vi "demo.vi"(0 "reference (in)":refnum<class "_Controller.lvclass">, 1 "position ref":refnum<vi>, 2 "position (large) ref":refnum<vi>, 5 "positions":i32[](array[numeric]), 11 "error in (no error)":errorcluster, 12 "status (display) ref":refnum<vi>, 13 "status ref":refnum<vi>) -> (4 "reference (out)":refnum<class "_Controller.lvclass">, 15 "error out":errorcluster)   [LabVIEW 2013, in "common.lvlib"]
doc: "Cycles the motor to each position in the input array of positions.\n\nProduced By:\n\n<B>Kod Integrations, LLC</B>\n4835 Marianne Drive\nMount Airy, MD 21771\nhttp://www.kodintegrations.com\nemail: info@kodintegrations.com\nphone: (240) 687-1288"
uses:
  libraries/common.lvlib
  controls/motor_status.ctl
  classes/Controller/_Controller.lvclass
  controls/axis.ctl
  controls/movement_item.ctl
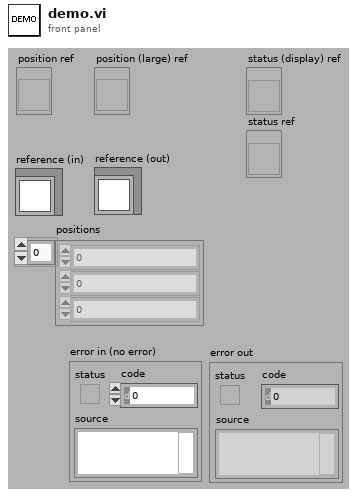
[diagram p1: front panel]
types:
  T1 = typedef "common.lvlib/movement_item.ctl" = cluster{"axis":T2, "target":i32}
  T2 = typedef "common.lvlib/axis.ctl" = enum16{"X", "Y", "Z", "U"}
  T3 = typedef "common.lvlib/motor_status.ctl" = enum16{"IDLE", "CONST", "ACCEL", "DECEL", "HOME_SWITCH", "-LIMIT_SWITCH", "+LIMIT_SWITCH", "-LIMIT_ERR", "+LIMIT_ERR", "COMM_TIMEOUT", "ALARM_INPUT", "ALARM_ERROR", "TOC_TIMEOUT_STATUS", "LATCH_INPUT_STATUS", "Z_INDEX_STATUS"}
  T4 = typedef "common.lvlib/complete_motor_state.ctl" = cluster{"X":T5, "Y":T5, "Z":T5, "U":T5, "buffer_enabled?":bool, "buffer_start":i32, "buffer_end":i32, "avail_buffer":i32, "move_mode":T6}
  T5 = typedef "common.lvlib/single_axis_state.ctl" = cluster{"motion_state":T3, "other_states":T3[]}
  T6 = typedef "common.lvlib/move_mode.ctl" = enum16{"ABSOLUTE", "INCREMENTAL"}
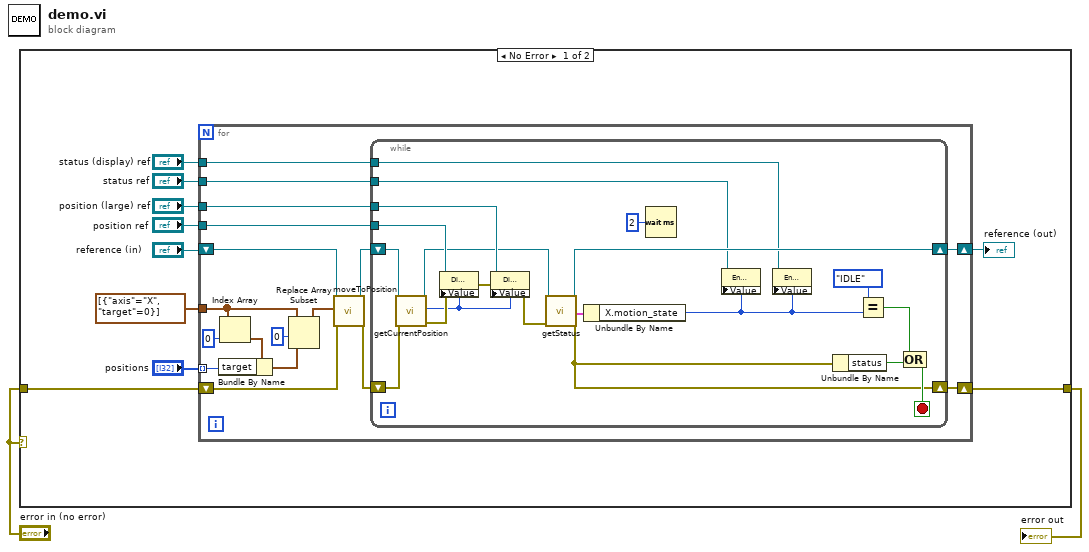
[diagram p0: block diagram]
diagram:
  n1 = case shown="No Error" "error in (no error)" {
    tunnel: "error in (no error)" -> [w8 w50]
    tunnel: [w7 w50] -> w1
    frame No Error {
      n2 = for {
        shift-right: [w23] -> w7
        shift-left: w8 -> [w24]
        tunnel: "positions" -> [w17] mode=indexing
        shift-right: [w27] -> w9
        shift-left: "reference (in)" -> [w29]
        tunnel: "position ref" -> [w26]
        tunnel: "position (large) ref" -> [w22]
        tunnel: "status (display) ref" -> [w21]
        tunnel: "status ref" -> [w20]
        tunnel: T1[] [{"axis"=enum."X", "target"=0}] ("target(s) (in)") -> [w16]
        n3 = Index Array(array=w16, index=0) -> (element=w18:T1)
        n4 = Bundle By Name(cluster=w18, "target"=w17) -> (w14:T1)
        n5 = Replace Array Subset(array=w16, new element=w14, index=0) -> (w13:T1[])
        n6 = call-dynamic "moveToPosition.vi"("Controller in"=w29, "target(s) (in)"=w13, "error in (no error)"=w24) -> ("Controller out"=w28:refnum<class "_Controller.lvclass">, "error out"=w25:errorcluster)  [unwired: 13 in, 2 out]
        n7 = while {
          shift-right: [w48] -> w27
          shift-left: w28 -> [w42]
          tunnel: w26 -> [w45]
          shift-right: [w41] -> w23
          shift-left: w25 -> [w44]
          tunnel: w22 -> [w39]
          tunnel: w21 -> [w36]
          tunnel: w20 -> [w35]
          stop <- w46 stop-if-true
          n8 = call-dynamic "getCurrentPosition.vi"("reference (in)"=w42, "error in (no error)"=w44) -> ("reference (out)"=w34:refnum<class "_Controller.lvclass">, "current_position (units)"=w33:i32, "error out"=w43:errorcluster)  [unwired: 15 in]
          n9 = property class="DigNum (strict)"(reference=w45, error in=w43, "Value"=w33) -> (error out=w38:errorcluster)  [unwired: 1 out]
          n10 = property class="DigNum (strict)"(reference=w39, error in=w38, "Value"=w33) -> (error out=w37:errorcluster)  [unwired: 1 out]
          n11 = call-dynamic "getStatus.vi"("reference (in)"=w34, "error in (no error)"=w37) -> ("reference (out)"=w48:refnum<class "_Controller.lvclass">, "full_state"=w32:T4, "error out"=w41:errorcluster)  [unwired: 14 in, 1 out]
          n12 = Unbundle By Name(w32) -> ("X.motion_state"=w30:T3)
          n13 = Wait (ms)(milliseconds to wait=u32 2) -> ()  [unwired: 1 out]
          n14 = property class="Enum (strict)"(reference=w35, "Value"=w30) -> ()  [unwired: 1 in, 2 out]
          n15 = property class="Enum (strict)"(reference=w36, "Value"=w30) -> ()  [unwired: 1 in, 2 out]
          n16 = Unbundle By Name(w41) -> ("status"=w47:bool)
          n17 = Equal?(x=motor_status."IDLE" ("X.motion_state"), y=w30) -> (x = y?=w40:bool)
          n18 = Compound Arithmetic op=OR(w40, w47) -> (w46:bool)
        }
      }
      "reference (out)" <- w9
    }
    frame Error {
    }
  }
  "error out" <- w1
